vi "YABOIJUAN.vi"(3 "NXT/EV3 2":T1) -> (0 "NXT/EV3 3":T1)   [LabVIEW 2016]
uses:
  <vilib>/NXT/Subs/LVHSConnector.ctl
  <vilib>/NXT/LegoClasses/BrickReference/BrickReference.lvclass
  <vilib>/NXT/Block Support/NXT_OutputPort.ctl
  <vilib>/NXT/Dual Mode Library/Display/clearDisplay.vi
  <vilib>/NXT/Dual Mode Library/Waits/Wait_Num.vi
  <vilib>/NXT/Dual Mode Library/Display/drawText.vi
  <vilib>/NXT/NXTIO Xnodes/NXTIONodeSubVIs/NXTMotorRunDistance.vi
  <vilib>/NXT/NXTIO Xnodes/AddressXNode/NXTIOAddress.xnode
  <vilib>/NXT/NXTIO Xnodes/NXTIOXNode/NXTIO.xnode
panel:
  out "Marble ID":dbl
  # "New Order\n\n0 BL\n1 RL\n2 BS\n3 RS\n4 HDPE\n5 WL\n6 Steel\n7 WS\n8 trash"
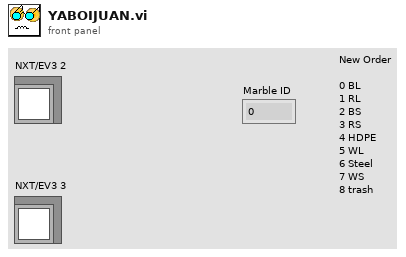
[diagram p1: front panel]
types:
  T1 = typedef "LVHSConnector.ctl" = refnum<class "BrickReference.lvclass">
  T2 = typedef "NXT_OutputPort.ctl" = u8
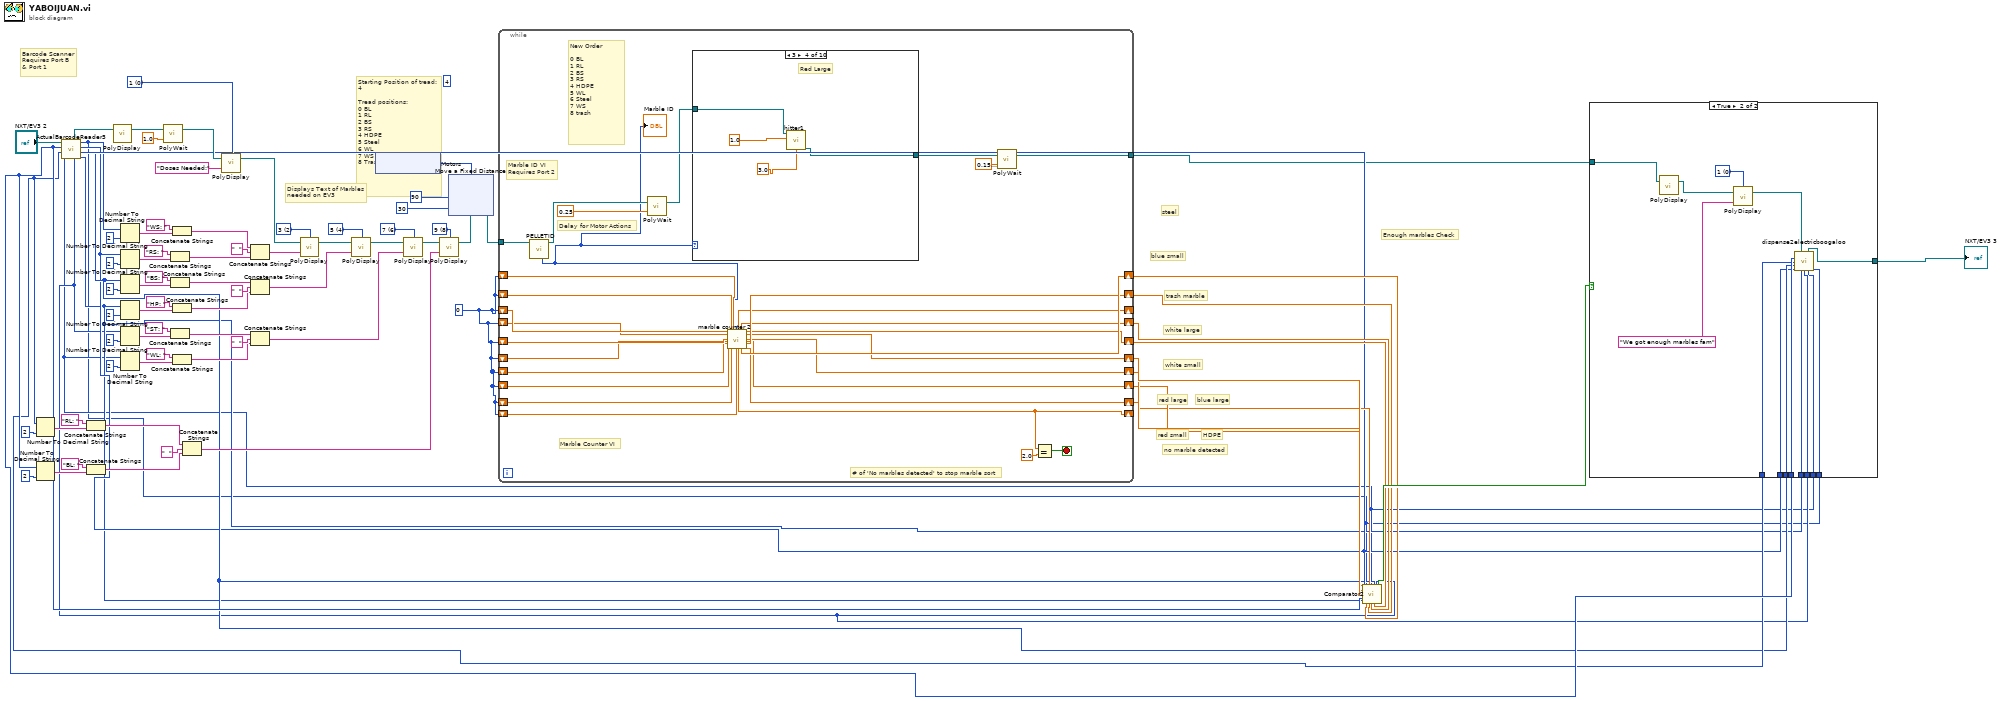
[diagram p0: block diagram]
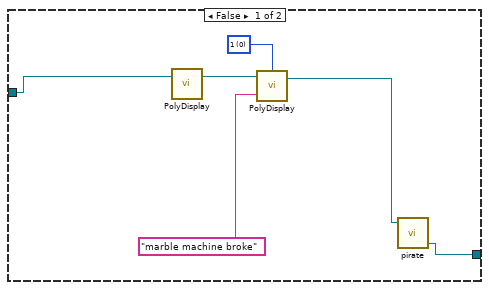
[diagram p2: hidden frame]
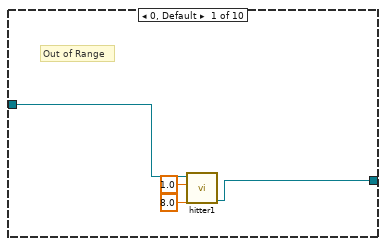
[diagram p3: hidden frame]
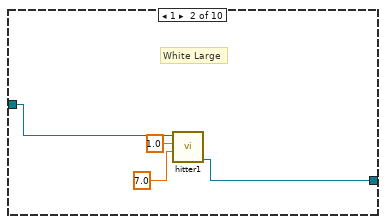
[diagram p4: hidden frame]
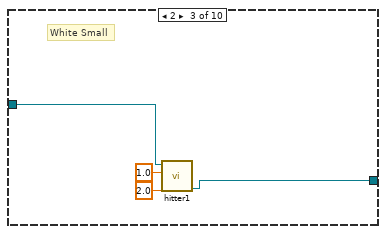
[diagram p5: hidden frame]
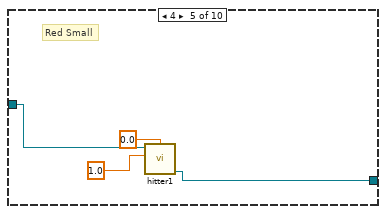
[diagram p6: hidden frame]
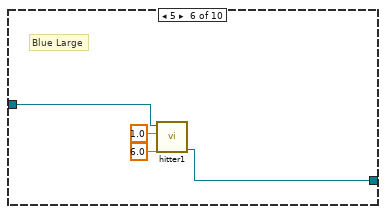
[diagram p7: hidden frame]
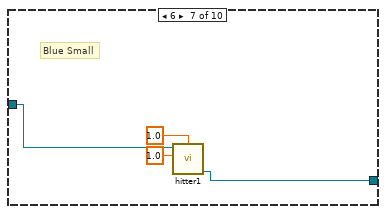
[diagram p8: hidden frame]
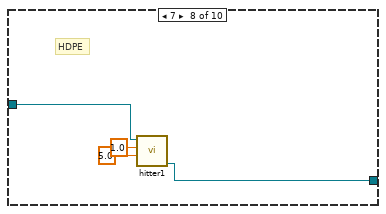
[diagram p9: hidden frame]
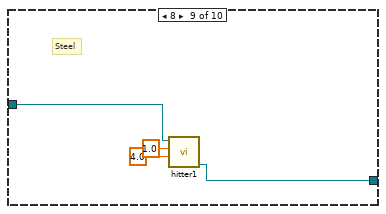
[diagram p10: hidden frame]
diagram:
  w24 = 0
  (unwired) 4
  w30 = i16 0 items=["1", "2", "3", "4", "5", "6", "7", "8", "9", "10", "11", "12"] ("Line")
  w51 = i16 4 items=["1", "2", "3", "4", "5", "6", "7", "8", "9", "10", "11", "12"] ("Line")
  w52 = i16 6 items=["1", "2", "3", "4", "5", "6", "7", "8", "9", "10", "11", "12"] ("Line")
  w53 = i16 2 items=["1", "2", "3", "4", "5", "6", "7", "8", "9", "10", "11", "12"] ("Line")
  w54 = i16 8 items=["1", "2", "3", "4", "5", "6", "7", "8", "9", "10", "11", "12"] ("Line")
  # "Enough marbles Check"
  # "no marble detected"
  # "HDPE"
  # "blue large"
  # "red small"
  # "red large"
  # "white small"
  # "white large"
  # "trash marble"
  # "blue small"
  # "steel"
  # "Starting Position of tread:\n4\n\nTread positions:\n0 BL\n1 RL\n2 BS\n3 RS\n4 HDPE\n5 Steel\n6 WL\n7 WS\n8 Trash"
  # "Displays Text of Marbles\nneeded on EV3"
  # "Barcode Scanner\nRequires Port B\n& Port 1"
  n1 = call "ActualBarcodeReader3.vi"("NXT/EV3"="NXT/EV3 2") -> ("O HPE"=w10:i32, "Blue Small"=w12:i32, "Red Small"=w11:i32, "White Small"=w7:i32, "Steel"=w9:i32, "NXT/EV3 2"=w25:T1, "White Large"=w8:i32, "Red Large"=w13:i32, "Blue Large"=w14:i32)  [unwired: 2 in]
  n2 = Number To Decimal String(number=w13, width (-)=i16 2) -> (decimal integer string=w57:string)
  n3 = Number To Decimal String(number=w14, width (-)=i16 2) -> (decimal integer string=w55:string)
  n4 = Concatenate Strings("RL: " ("string"), w57) -> (w40:string)
  n5 = Concatenate Strings("BL: " ("string"), w55) -> (w39:string)
  n6 = call-poly <vilib>:"PolyDisplay.vi"("NXT/EV3"=w25) -> ("NXT/EV3"=w80:T1)  [unwired: 3 in]
  n7 = Number To Decimal String(number=w7, width (-)=i16 2) -> (decimal integer string=w70:string)
  n8 = Number To Decimal String(number=w11, width (-)=i16 2) -> (decimal integer string=w67:string)
  n9 = Number To Decimal String(number=w12, width (-)=i16 2) -> (decimal integer string=w65:string)
  n10 = Number To Decimal String(number=w10, width (-)=i16 2) -> (decimal integer string=w63:string)
  n11 = Number To Decimal String(number=w9, width (-)=i16 2) -> (decimal integer string=w61:string)
  n12 = Number To Decimal String(number=w8, width (-)=i16 2) -> (decimal integer string=w59:string)
  n13 = call-poly <vilib>:"PolyWait.vi"("Time (1 sec)"=sgl 1.0, "NXT/EV3"=w80) -> ("NXT/EV3"=w29:T1)  [unwired: 2 in]
  n14 = Concatenate Strings("RS: " ("string"), w67) -> (w48:string)
  n15 = Concatenate Strings("BS: " ("string"), w65) -> (w44:string)
  n16 = Concatenate Strings("ST: " ("string"), w61) -> (w42:string)
  n17 = Concatenate Strings("HP: " ("string"), w63) -> (w43:string)
  n18 = Concatenate Strings("WS: " ("string"), w70) -> (w50:string)
  n19 = Concatenate Strings("WL: " ("string"), w59) -> (w41:string)
  n20 = Concatenate Strings(w40, "  " ("string"), w39) -> (w35:string)
  n21 = call-poly <vilib>:"PolyDisplay.vi"("Text"="Doses Needed:", "NXT/EV3"=w29, "Line"=w30) -> ("NXT/EV3"=w28:T1)  [unwired: 1 in]
  n22 = Concatenate Strings(w50, "  " ("string"), w48) -> (w38:string)
  n23 = Concatenate Strings(w44, "  " ("string"), w43) -> (w37:string)
  n24 = Concatenate Strings(w42, "  " ("string"), w41) -> (w36:string)
  n25 = call-poly <vilib>:"PolyDisplay.vi"("Text"=w38, "NXT/EV3"=w28, "Line"=w53) -> ("NXT/EV3"=w34:T1)  [unwired: 1 in]
  n26 = call-poly <vilib>:"PolyDisplay.vi"("Text"=w37, "NXT/EV3"=w34, "Line"=w51) -> ("NXT/EV3"=w33:T1)  [unwired: 1 in]
  n27 = xnode "Motors"() -> ("Motor"=w3:T2)
  n28 = call-poly <vilib>:"PolyDisplay.vi"("Text"=w36, "NXT/EV3"=w33, "Line"=w52) -> ("NXT/EV3"=w32:T1)  [unwired: 1 in]
  n29 = call-poly <vilib>:"PolyDisplay.vi"("Text"=w35, "NXT/EV3"=w32, "Line"=w54) -> ("NXT/EV3"=w5:T1)  [unwired: 1 in]
  n30 = xnode "Move a Fixed Distance"("Speed 1"=i8 30, "Distance 1"=90, "Motors"=w3, "NXT/EV3"=w5) -> ("NXT/EV3"=w4:T1)
  n31 = while {
    tunnel: w4 -> [w108]
    shift-right: [w103] -> w22
    shift-left: w24 -> [w104]
    shift-right: [w101] -> w21
    shift-left: w24 -> [w102]
    shift-right: [w99] -> _
    shift-left: w24 -> [w100]
    shift-right: [w97] -> w20
    shift-left: w24 -> [w98]
    shift-right: [w95] -> w19
    shift-left: w24 -> [w96]
    shift-right: [w93] -> w18
    shift-left: w24 -> [w94]
    shift-right: [w91] -> w17
    shift-left: w24 -> [w92]
    shift-right: [w89] -> w16
    shift-left: w24 -> [w90]
    shift-right: [w87] -> w15
    shift-left: w24 -> [w88]
    shift-right: [w85] -> _
    shift-left: w24 -> [w86]
    tunnel: [w83] -> w6
    stop <- w105 stop-if-true
    # "New Order\n\n0 BL\n1 RL\n2 BS\n3 RS\n4 HDPE\n5 WL\n6 Steel\n7 WS\n8 trash"
    # "# of 'No marbles detected' to stop marble sort"
    # "Marble Counter VI"
    # "Delay for Motor Actions"
    # "Marble ID VI\nRequires Port 2"
    n32 = call "PELLETID.vi"("NXT/EV3"=w108) -> ("Marble ID#"=w81:i32, "NXT/EV3 2"=w107:T1)  [unwired: 8 in]
    "Marble ID" <- w81
    n33 = call-poly <vilib>:"PolyWait.vi"("Time (1 sec)"=sgl 0.25, "NXT/EV3"=w107) -> ("NXT/EV3"=w109:T1)  [unwired: 2 in]
    n34 = case shown="3" w81 {
      tunnel: w109 -> [w114 w118 w122 w125 w130 w133 w138 w141 w145 w147]
      tunnel: [w113 w117 w119 w126 w129 w134 w137 w142 w146 w147] -> w84
      frame 0, Default {
        # "Out of Range"
        n35 = call "hitter1.vi"("increments"=8.0, "+ or -"=1.0, "NXT/EV3"=w114) -> ("NXT/EV3 2"=w113:T1)
      }
      frame 1 {
        # "White Large"
        n36 = call "hitter1.vi"("increments"=7.0, "+ or -"=1.0, "NXT/EV3"=w118) -> ("NXT/EV3 2"=w117:T1)
      }
      frame 2 {
        # "White Small"
        n37 = call "hitter1.vi"("increments"=2.0, "+ or -"=1.0, "NXT/EV3"=w122) -> ("NXT/EV3 2"=w119:T1)
      }
      frame 3 {
        # "Red Large"
        n38 = call "hitter1.vi"("increments"=3.0, "+ or -"=1.0, "NXT/EV3"=w125) -> ("NXT/EV3 2"=w126:T1)
      }
      frame 4 {
        # "Red Small"
        n39 = call "hitter1.vi"("increments"=0.0, "+ or -"=1.0, "NXT/EV3"=w130) -> ("NXT/EV3 2"=w129:T1)
      }
      frame 5 {
        # "Blue Large"
        n40 = call "hitter1.vi"("increments"=6.0, "+ or -"=1.0, "NXT/EV3"=w133) -> ("NXT/EV3 2"=w134:T1)
      }
      frame 6 {
        # "Blue Small"
        n41 = call "hitter1.vi"("increments"=1.0, "+ or -"=1.0, "NXT/EV3"=w138) -> ("NXT/EV3 2"=w137:T1)
      }
      frame 7 {
        # "HDPE"
        n42 = call "hitter1.vi"("increments"=5.0, "+ or -"=1.0, "NXT/EV3"=w141) -> ("NXT/EV3 2"=w142:T1)
      }
      frame 8 {
        # "Steel"
        n43 = call "hitter1.vi"("increments"=4.0, "+ or -"=1.0, "NXT/EV3"=w145) -> ("NXT/EV3 2"=w146:T1)
      }
      frame 9 {
        # "No Marble Detected"
      }
    }
    n44 = call "marble counter 2.vi"("Trash Marble-in"=w100, "White Large-in"=w98, "White Small-in"=w96, "Red Large-in"=w94, "Red small-in"=w92, "Blue Large-in"=w90, "blue small-in"=w102, "HDPE-in"=w88, "Steel -in"=w104, "Marble Type Input"=w81, "No marble Detected-in"=w86) -> ("Trash Marble-out"=w99:dbl, "No marble Detected-out"=w85:dbl, "White Large-out"=w97:dbl, "Steel-out"=w103:dbl, "White small-out"=w95:dbl, "Red Large-out"=w93:dbl, "Red small-out"=w91:dbl, "blue large-out"=w89:dbl, "blue small-out"=w101:dbl, "HDPE-out"=w87:dbl)  [unwired: 7 in]
    n45 = call-poly <vilib>:"PolyWait.vi"("Time (1 sec)"=sgl 0.15, "NXT/EV3"=w84) -> ("NXT/EV3"=w83:T1)  [unwired: 2 in]
    n46 = Equal?(x=w85, y=2.0) -> (x = y?=w105:bool)
  }
  n47 = call "Comparator2.vi"("7-have"=w16, "5-code"=w13, "6-have"=w17, "6-code"=w11, "5- have"=w18, "7-code"=w14, "8-code"=w10, "4-code"=w7, "1-have"=w22, "8-have"=w15, "2-have"=w21, "3 - code"=w8, "3- have"=w20, "2-code"=w12, "4-have"=w19, "1 - code"=w9) -> ("Enough Marbles?"=w23:bool)  [unwired: 11 in]
  n48 = case shown="True" w23 {
    tunnel: [w149 w164] -> w27
    tunnel: w14 -> [_ w162]
    tunnel: w13 -> [_ w161]
    tunnel: w12 -> [_ w160]
    tunnel: w11 -> [_ w159]
    tunnel: w10 -> [_ w158]
    tunnel: w9 -> [_ w157]
    tunnel: w8 -> [_ w156]
    tunnel: w7 -> [_ w155]
    tunnel: w6 -> [w148 w154]
    frame False {
      w151 = i16 0 items=["1", "2", "3", "4", "5", "6", "7", "8", "9", "10", "11", "12"] ("Line")
      n49 = call-poly <vilib>:"PolyDisplay.vi"("NXT/EV3"=w148) -> ("NXT/EV3"=w153:T1)  [unwired: 3 in]
      n50 = call-poly <vilib>:"PolyDisplay.vi"("Text"="marble machine broke", "NXT/EV3"=w153, "Line"=w151) -> ("NXT/EV3"=w150:T1)  [unwired: 1 in]
      n51 = call "pirate.vi"("NXT/EV3"=w150) -> ("NXT/EV3 2"=w149:T1)  [unwired: 1 in]
    }
    frame True {
      w165 = i16 0 items=["1", "2", "3", "4", "5", "6", "7", "8", "9", "10", "11", "12"] ("Line")
      n52 = call-poly <vilib>:"PolyDisplay.vi"("NXT/EV3"=w154) -> ("NXT/EV3"=w167:T1)  [unwired: 3 in]
      n53 = call-poly <vilib>:"PolyDisplay.vi"("Text"="We got enough marbles fam", "NXT/EV3"=w167, "Line"=w165) -> ("NXT/EV3"=w163:T1)  [unwired: 1 in]
      n54 = call "dispense2electricboogaloo.vi"("NXT/EV3"=w163, "0-Blue Large"=w162, "1-Red Large"=w161, "2-Blue Small"=w160, "3-Red Small"=w159, "4-HDPE"=w158, "5-Steel"=w157, "6-White Large"=w156, "7-White Small"=w155) -> ("NXT/EV3 2"=w164:T1)  [unwired: 6 in]
    }
  }
  "NXT/EV3 3" <- w27
